vi "TestAll.vi"(8 "error in (no error)":errorcluster, 10 "No. of Runs":i32=1, 11 "Test Cases":bool[](array[boolean])=[FALSE, FALSE, FALSE]) -> (0 "error out":errorcluster, 3 "report":string)   [LabVIEW 2018]
uses:
  <vilib>/addons/_JKI Toolkits/Caraya/classes/Test Suite/Define Test Suite (SimpleText Report).vi
  <vilib>/addons/_JKI Toolkits/Caraya/classes/Test Suite/Test Suite.lvclass
panel:
  out "Succeeded?":bool
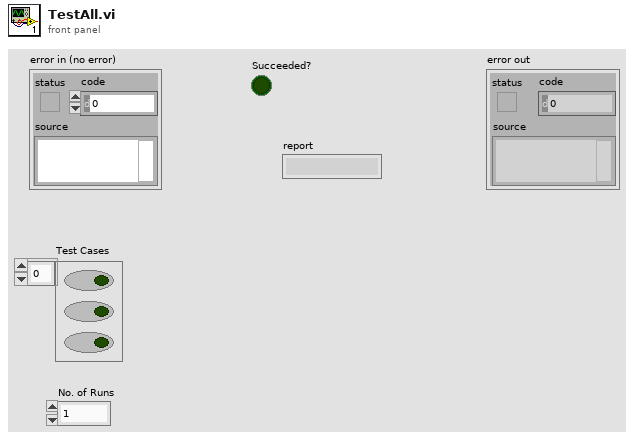
[diagram p1: front panel]
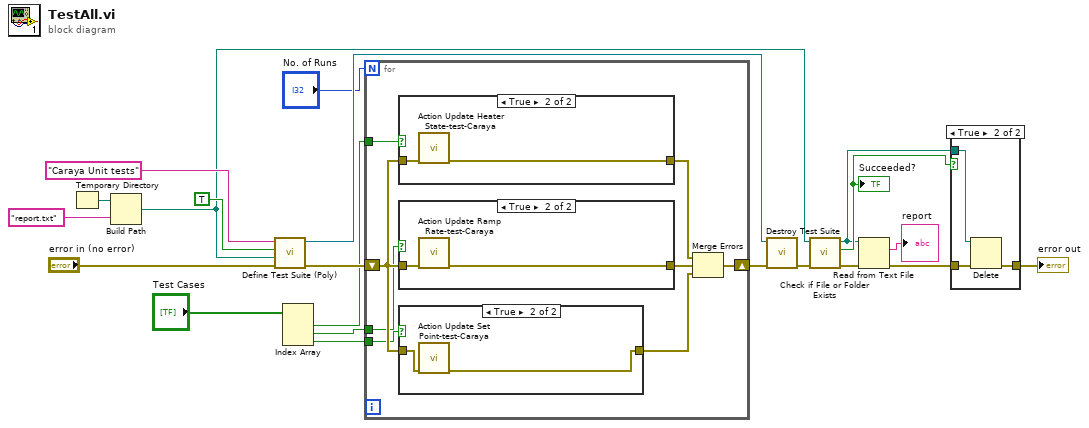
[diagram p0: block diagram]
diagram:
  n1 = Temporary Directory() -> (w17:path)
  n2 = Build Path(base path=w17, name or relative path="report.txt") -> (appended path=w11:path)
  n3 = call-poly <vilib>:"Define Test Suite (Poly).vi"("error in (no error)"="error in (no error)", "Report Path"=w11, "Interactive"=TRUE, "Label (VI Title)"="Caraya Unit tests") -> ("error out"=w7:errorcluster, "Test Suite"=w19:refnum<class "Test Suite.lvclass">)  [unwired: 6 in]
  n4 = Index Array(array="Test Cases") -> (element #1=w5:bool, element #2=w4:bool, element #3=w3:bool)  [unwired: 3 in]
  n5 = for {
    N: "No. of Runs" -> [_]
    tunnel: w5 -> [w24]
    tunnel: w4 -> [w23]
    tunnel: w3 -> [w22]
    shift-right: [w29] -> w10
    shift-left: w7 -> [w26]
    n6 = case shown="True" w24 {
      tunnel: w26 -> [w36 w38]
      tunnel: [w36 w37] -> w28
      frame False {
      }
      frame True {
        n7 = call "Action Update Heater State-test-Caraya.vi"("error in (no error)"=w38) -> ("error out"=w37:errorcluster)  [unwired: 10 in]
      }
    }
    n8 = case shown="True" w23 {
      tunnel: w26 -> [w33 w35]
      tunnel: [w33 w34] -> w27
      frame False {
      }
      frame True {
        n9 = call "Action Update Ramp Rate-test-Caraya.vi"("error in (no error)"=w35) -> ("error out"=w34:errorcluster)  [unwired: 10 in]
      }
    }
    n10 = case shown="True" w22 {
      tunnel: w26 -> [w30 w32]
      tunnel: [w30 w31] -> w25
      frame False {
      }
      frame True {
        n11 = call "Action Update Set Point-test-Caraya.vi"("error in (no error)"=w32) -> ("error out"=w31:errorcluster)  [unwired: 10 in]
      }
    }
    n12 = Merge Errors(w28, w27, w25) -> (w29:errorcluster)
  }
  n13 = call-dynamic "Destroy Test Suite.vi"("error in (no error)"=w10, "Test Suite in"=w19) -> ("error out"=w2:errorcluster)  [unwired: 9 in]
  n14 = call <vilib>:"Check if File or Folder Exists.vi"("error in (no error)"=w2, "path"=w11) -> ("error out"=w14:errorcluster, "file or folder exists?"=w15:bool, "dup path"=w12:path)  [unwired: 7 in]
  "Succeeded?" <- w15
  n15 = Read from Text File(file (use dialog)=w12, error in=w14) -> (text=→"report":string, error out=w13:errorcluster)  [unwired: 2 in, 2 out]
  n16 = case shown="True" w15 {
    tunnel: w12 -> [_ w42]
    tunnel: w13 -> [w39 w41]
    tunnel: [w39 w40] -> w9
    frame False {
    }
    frame True {
      n17 = Delete(path (use dialog)=w42, error in=w41) -> (error out=w40:errorcluster)  [unwired: 3 in, 2 out]
    }
  }
  "error out" <- w9
